vi "Configure Measurement Window.vi"(8 "error in (no error)":errorcluster {"code" format="%.0x"}, 9 "Window Type (1:Rectangular)":u16(ring)=1 items=["Hanning", "Rectangular"], 10 "Channel Name (1)":string="1", 11 "VISA resource name":refnum<visa-resource-name>) -> (0 "error out":errorcluster {"code" format="%.0x"}, 3 "VISA resource name out":refnum<visa-resource-name>)   [LabVIEW 2014, in "Agilent N6700 Series.lvlib"]
doc: "Sets a signal conditioning function used in DC measurement calculations on models that have measurement controls.\n\n<b>Note:</b>\nThis VI only applies to models N676xA, N678xA SMU, or models N673xA. N674xA, N675xA, and N677xA with Option 054 (High Speed Test Extensions)."
uses:
  Agilent N6700 Series.lvlib
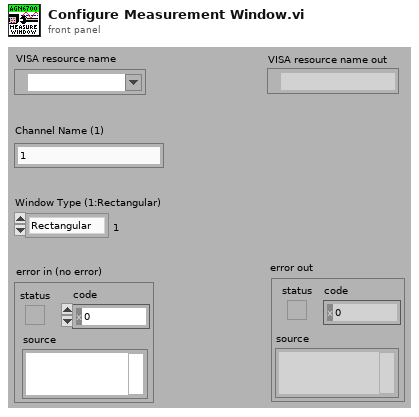
[diagram p1: front panel]
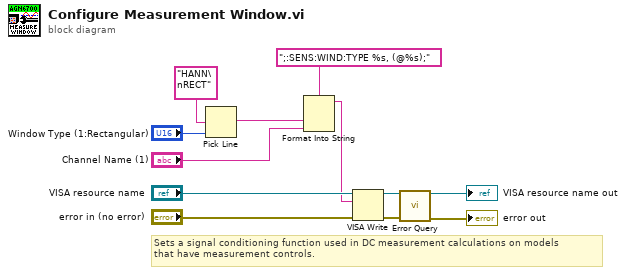
[diagram p0: block diagram]
diagram:
  # "Sets a signal conditioning function used in DC measurement calculations on models \nthat have measurement controls."
  n1 = Pick Line(multi-line string="HANN\nRECT", line index="Window Type (1:Rectangular)") -> (output string=w1:string)  [unwired: 1 in]
  n2 = Format Into String(format string=";:SENS:WIND:TYPE %s, (@%s);", w1, "Channel Name (1)") -> (resulting string=w4:string)  [unwired: 2 in, 1 out]
  n3 = VISA Write(VISA resource name="VISA resource name", write buffer=w4, error in (no error)="error in (no error)") -> (VISA resource name out=w8:refnum<visa-resource-name>, error out=w7:errorcluster)  [unwired: 1 out]
  n4 = call "Error Query.vi"("VISA resource name"=w8, "error in (no error)"=w7) -> ("VISA resource name out"=→"VISA resource name out":refnum<visa-resource-name>, "error out"=→"error out":errorcluster)  [unwired: 10 in, 2 out]
